vi "FT10_Connect Unitherm.vi"(8 "error in (no error)":errorcluster, 11 "Message Handling Cluster in":T1) -> (0 "error out":errorcluster, 3 "Message Handling Cluster out":T1)   [LabVIEW 2024]
doc: "Establishes a VISA connection with the Unitherm hardware.\nUnitherm simulates resistance loads for testing generator."
uses:
  Controls/Control_Message Handling Cluster.ctl
  Controls/Control_M4X Connection.ctl
  <vilib>/Instr/_visa.llb/VISA Configure Serial Port (Instr).vi
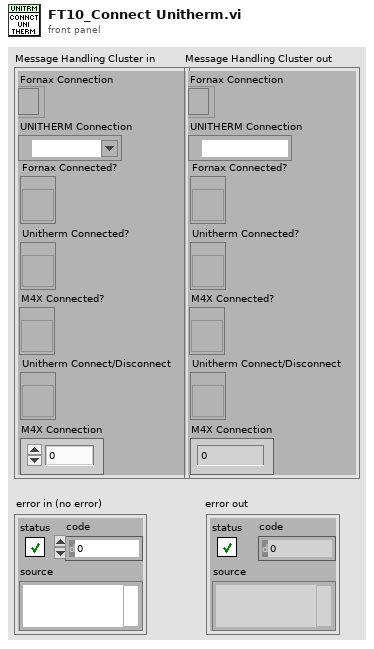
[diagram p1: front panel]
types:
  T1 = typedef "Control_Message Handling Cluster.ctl" = cluster{"Fornax Connection":refnum<k5>, "UNITHERM Connection":refnum<visa-resource-name>, "Fornax Connected?":refnum<vi>, "Unitherm Connected?":refnum<vi>, "M4X Connected?":refnum<vi>, "Unitherm Connect/Disconnect":refnum<vi>, "M4X Connection":T2}
  T2 = typedef "Control_M4X Connection.ctl" = u32
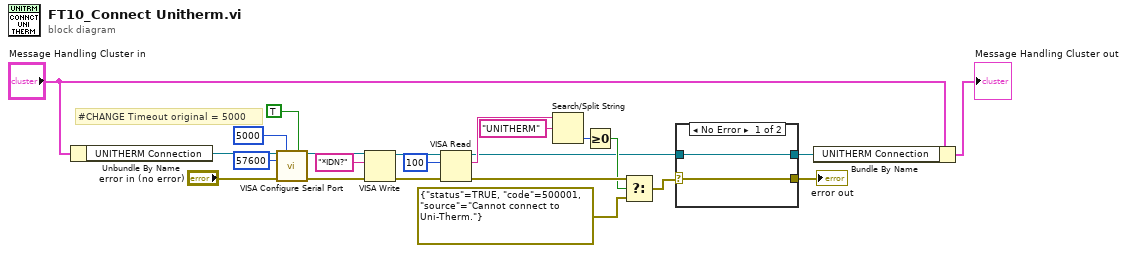
[diagram p0: block diagram]
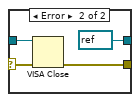
[diagram p2: hidden frame]
diagram:
  # "#CHANGE Timeout original = 5000"
  n1 = Unbundle By Name("Message Handling Cluster in") -> ("UNITHERM Connection"=w3:refnum<visa-resource-name>)
  n2 = call-poly "VISA Configure Serial Port"("VISA resource name"=w3, "timeout (10sec)"=u32 5000, "Enable Termination\nChar (T)"=TRUE ("Enable Termination\nChar (T)"), "baud rate (9600)"=u32 57600, "error in (no error)"="error in (no error)") -> ("VISA resource name out"=w13:refnum<visa-resource-name>, "error out"=w14:errorcluster)  [unwired: 9 in]
  n3 = VISA Write(VISA resource name=w13, write buffer="*IDN?" ("string"), error in (no error)=w14) -> (VISA resource name out=w9:refnum<visa-resource-name>, error out=w10:errorcluster)  [unwired: 1 out]
  n4 = VISA Read(VISA resource name=w9, byte count=u32 100, error in (no error)=w10) -> (VISA resource name out=w6:refnum<visa-resource-name>, read buffer=w18:string, error out=w23:errorcluster)  [unwired: 1 out]
  n5 = Search/Split String(string=w18, search string/char (-)="UNITHERM") -> (offset of match=w20:i32)  [unwired: 1 in, 2 out]
  n6 = Greater Or Equal To 0?(x=w20) -> (x >= 0?=w21:bool)
  n7 = Select(t=w23, s=w21, f=errorcluster {"status"=TRUE, "code"=500001, "source"="Cannot connect to Uni-Therm."} ("error constant")) -> (s? t:f=w7:errorcluster)
  n8 = case shown="No Error" w7 {
    selector: w7 -> [w24 w28]
    tunnel: w6 -> [w25 w26]
    tunnel: [w25 refnum<visa-resource-name> refnum ("VISA resource name out")] -> w2
    tunnel: [w24 w27] -> w5
    frame No Error {
    }
    frame Error {
      n9 = VISA Close(VISA resource name=w26, error in (no error)=w28) -> (error out=w27:errorcluster)
    }
  }
  "error out" <- w5
  n10 = Bundle By Name(cluster="Message Handling Cluster in", "UNITHERM Connection"=w2) -> (→"Message Handling Cluster out":T1)
